vi "Decode response.vi"(8 "error in":errorcluster, 10 "response in":string="$ID1,1.6,005842.1,1E26", 11 "F-70 parameters in":T1 {"Last updated" format="%<%d/%m/%Y %H:%M:%S>T"; "State of operation" items=["Local Off", "Local On", "Remote Off", "Remote On", "Cold head Run", "Cold head pause", "Fault Off", "Oil Fault Off"]; "Return pressure (PSIG)" scale=0.0..200.0; "Water in Tmp (°C)" scale=0.0..100.0; "Water out Tmp (°C)" scale=0.0..100.0; "He discharge Tmp (°C)" scale=0.0..100.0}) -> (0 "error out":errorcluster, 3 "F-70 parameters out":T1 {"Last updated" format="%<%d/%m/%Y %H:%M:%S>T"; "State of operation" items=["Local Off", "Local On", "Remote Off", "Remote On", "Cold head Run", "Cold head pause", "Fault Off", "Oil Fault Off"]; "Return pressure (PSIG)" scale=0.0..200.0; "Water in Tmp (°C)" scale=0.0..100.0; "Water out Tmp (°C)" scale=0.0..100.0; "He discharge Tmp (°C)" scale=0.0..100.0})   [LabVIEW 2021, in "F-70 driver.lvlib"]
doc: "Process response message and updates F-70 properties cluster by values and states.\n\nErrors:\nUnknown or unexpected comunication error occured -› Sent command, checksum or format of response is incorrect.\nInvalid command code -› Compressor received invalid message."
uses:
  <instrlib>/F-70 driver/F-70 driver.lvlib
  <instrlib>/F-70 driver/public/F-70 parameters.ctl
  <instrlib>/F-70 driver/public/Commands.ctl
  <vilib>/Utility/error.llb/Error Cluster From Error Code.vi
  <vilib>/ErrorRing/Error Ring.xnode
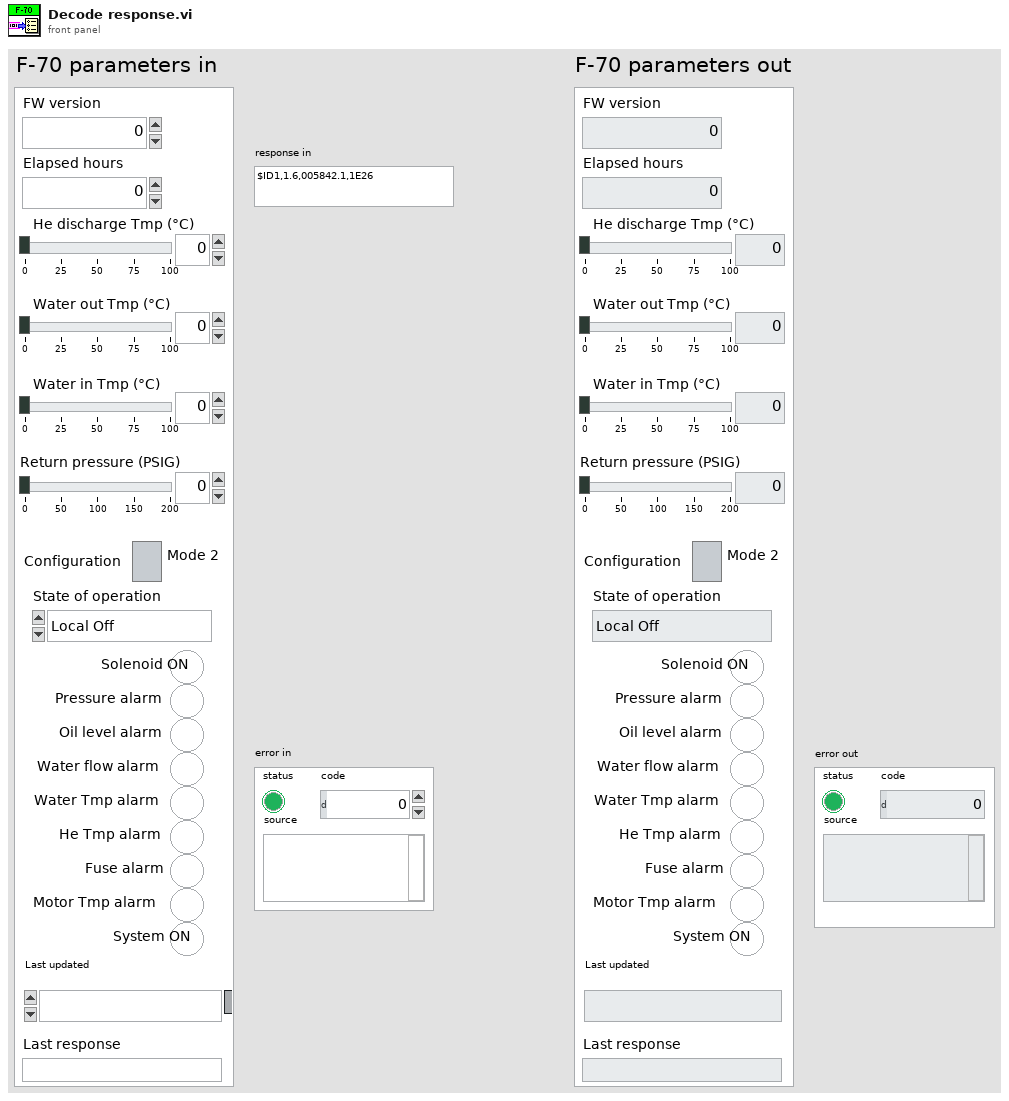
[diagram p1: front panel]
types:
  T1 = typedef "F-70 driver.lvlib/F-70 parameters.ctl" = cluster{"FW version":dbl, "Elapsed hours":dbl, "He discharge Tmp (°C)":dbl, "Water out Tmp (°C)":dbl, "Water in Tmp (°C)":dbl, "Return pressure (PSIG)":dbl, "Configuration":bool, "State of operation":u16, "Solenoid ON":bool, "Pressure alarm":bool, "Oil level alarm":bool, "Water flow alarm":bool, "Water Tmp alarm":bool, "He Tmp alarm":bool, "Fuse alarm":bool, "Motor Tmp alarm":bool, "System ON":bool, "Last updated":timestamp, "Last response":string}
  T2 = typedef "F-70 driver.lvlib/Commands.ctl" = enum16{"TEA", "PRA", "STA", "ID1", "ON1", "RS1", "CHP", "OFF", "CHR", "POF", "TE1", "TE2", "TE3", "TE4", "PR1", "PR2", "???"}
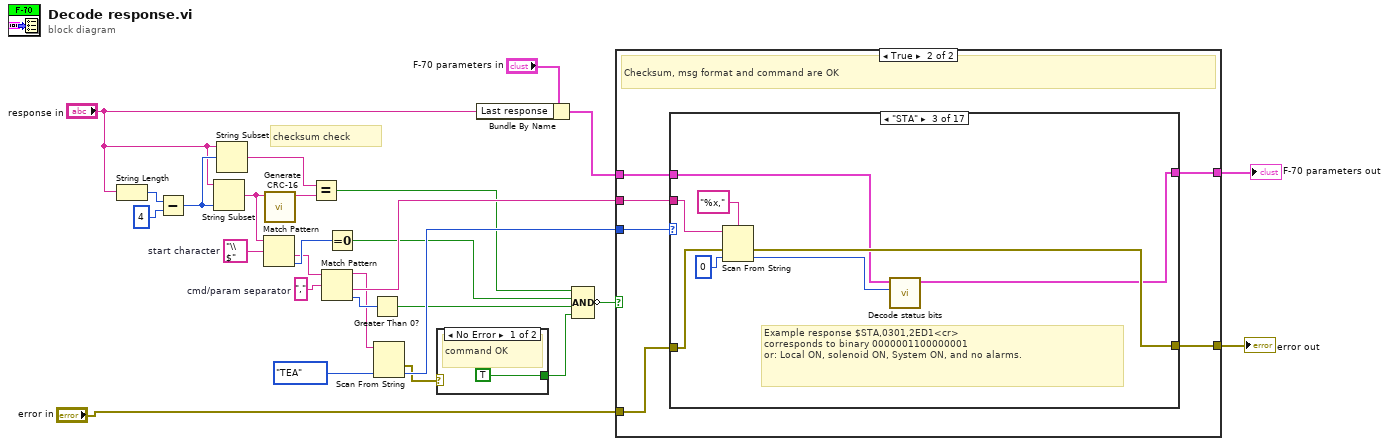
[diagram p0: block diagram]
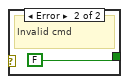
[diagram p2: hidden frame]
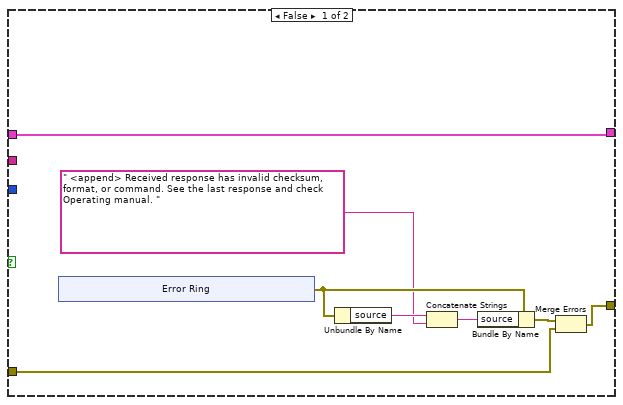
[diagram p3: hidden frame]
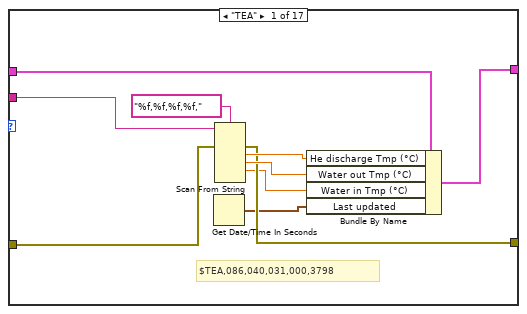
[diagram p4: hidden frame]
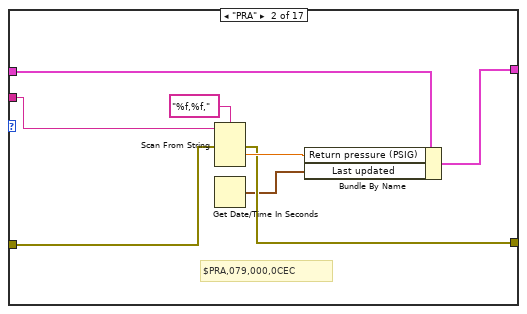
[diagram p5: hidden frame]
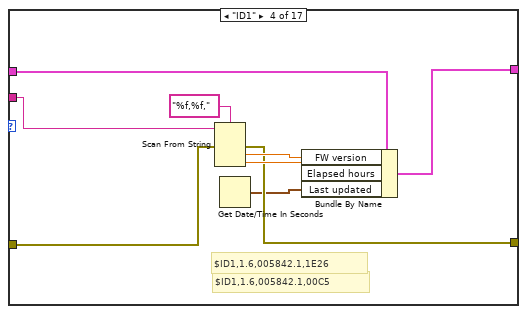
[diagram p6: hidden frame]
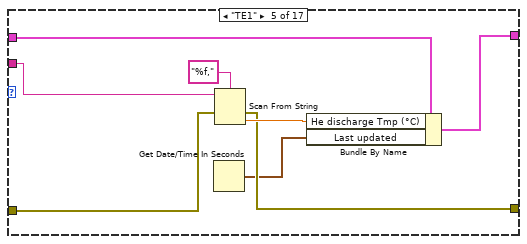
[diagram p7: hidden frame]
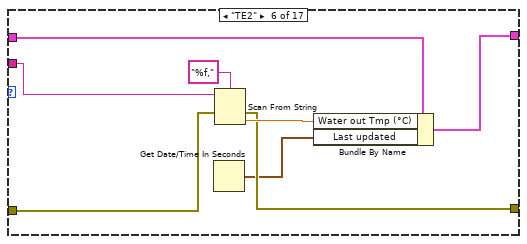
[diagram p8: hidden frame]
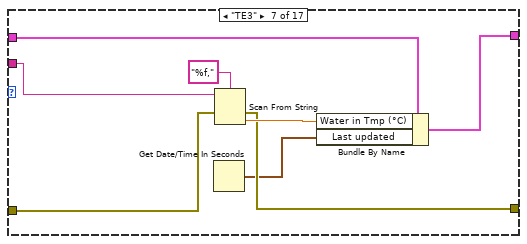
[diagram p9: hidden frame]
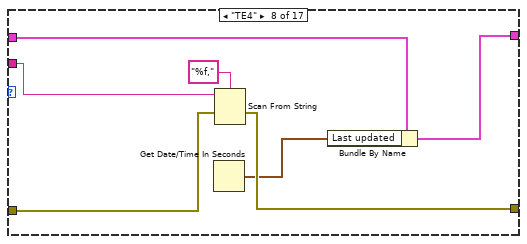
[diagram p10: hidden frame]
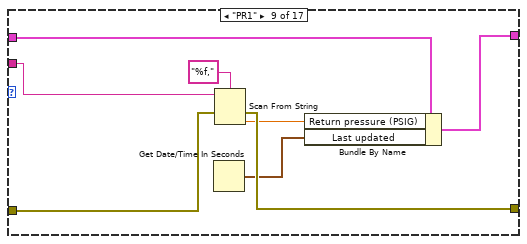
[diagram p11: hidden frame]
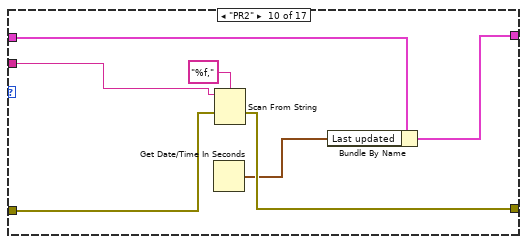
[diagram p12: hidden frame]
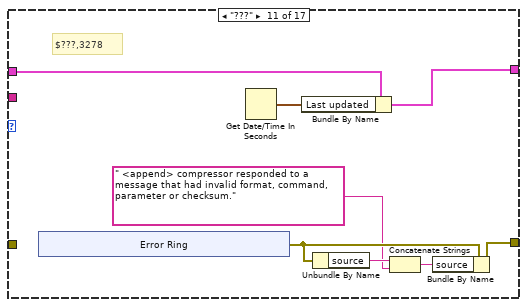
[diagram p13: hidden frame]
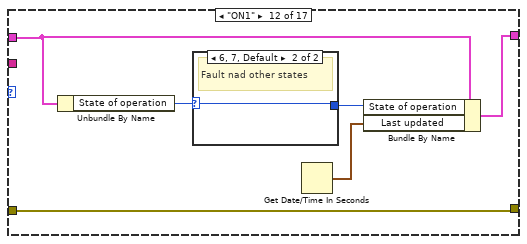
[diagram p14: hidden frame]
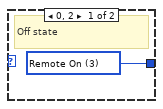
[diagram p15: hidden frame]
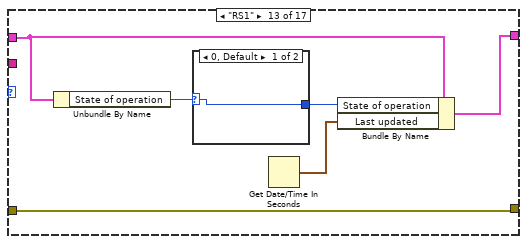
[diagram p16: hidden frame]
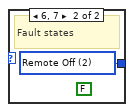
[diagram p17: hidden frame]
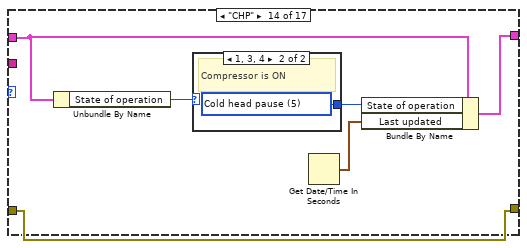
[diagram p18: hidden frame]
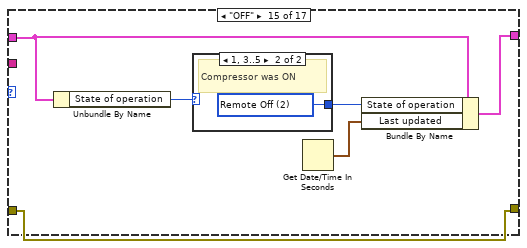
[diagram p20: hidden frame]
diagram:
  w16 = ","  # cmd/param separator
  w20 = "\\$"  # start character
  # "checksum check"
  n1 = String Length(string="response in") -> (length=w26:i32)
  n2 = Subtract(x=w26, y=4) -> (x-y=w24:i32)
  n3 = String Subset(string="response in", length (rest)=w24) -> (substring=w21:string)  [unwired: 1 in]
  n4 = String Subset(string="response in", offset (0)=w24) -> (substring=w11:string)  [unwired: 1 in]
  n5 = Match Pattern(string=w21, regular expression=w20) -> (after substring=w17:string, offset past match=w19:i32)  [unwired: 1 in, 2 out]
  n6 = call <instrlib>:"Generate CRC-16.vi"("DATA PACKET"=w21) -> ("CRC-16 H-str"=w10:string)  [unwired: 4 in, 2 out]
  n7 = Equal?(x=w11, y=w10) -> (x = y?=w8:bool)
  n8 = Match Pattern(string=w17, regular expression=w16) -> (before substring=w12:string, after substring=w15:string, offset past match=w18:i32)  [unwired: 1 in, 1 out]
  n9 = Equal To 0?(x=w19) -> (x = 0?=w4:bool)
  n10 = Greater Than 0?(x=w18) -> (x > 0?=w5:bool)
  n11 = Scan From String(input string=w12, default 1=Commands."TEA" ("Commands")) -> (error out=w1:errorcluster, output 1=w13:T2)  [unwired: 3 in, 2 out]
  n12 = case shown="No Error" w1 {
    tunnel: [TRUE FALSE] -> w3
    frame No Error {
      # "command OK"
    }
    frame Error {
      # "Invalid cmd"
    }
  }
  n13 = Bundle By Name(cluster="F-70 parameters in", "Last response"="response in") -> (w7:T1)
  n14 = Compound Arithmetic op=AND(w8, w4, w5, w3) -> (invert w9:bool)
  n15 = case shown="True" w9 {
    tunnel: [w32 w47] -> w27
    tunnel: "error in" -> [w31 w46]
    tunnel: [w33 w45] -> w22
    tunnel: w15 -> [_ w44]
    tunnel: w13 -> [_ w43]
    tunnel: w7 -> [w33 w42]
    frame False {
      n16 = xnode "Error Ring"() -> ("error out"=w35:errorcluster)
      n17 = Unbundle By Name(w35) -> ("source"=w36:string)
      n18 = Concatenate Strings(w36, " <append> Received response has invalid checksum, format, or command. See the last response and check Operating manual. " ("string")) -> (w37:string)
      n19 = Bundle By Name(cluster=w35, "source"=w37) -> (w34:errorcluster)
      n20 = Merge Errors(w34, w31) -> (w32:errorcluster)
    }
    frame True {
      # "Checksum, msg format and command are OK"
      n21 = case shown="\"STA\"" w43 {
        tunnel: [w51 w60 w71 w76 w85 w93 w101 w109 w117 w124 w133 w144 w152 w160 w168 w176 w181] -> w47
        tunnel: w46 -> [w52 w61 w72 w77 w86 w94 w102 w110 w118 w125 _ w144 w152 w160 w168 w176 w181]
        tunnel: w42 -> [w56 w64 w69 w81 w89 w97 w105 w112 w120 w127 w136 w143 w151 w159 w167 w175 w183]
        tunnel: [w53 w62 w68 w78 w87 w95 w103 w111 w119 w126 w135 w146 w154 w162 w170 w178 w182] -> w45
        tunnel: w44 -> [w48 w58 w66 w74 w83 w91 w99 w107 w114 w122 _ _ _ _ _ _ _]
        frame "TEA" {
          # "$TEA,086,040,031,000,3798"
          n22 = Get Date/Time In Seconds() -> (seconds since 1Jan1904=w50:timestamp)
          n23 = Scan From String(format string="%f,%f,%f,%f,", input string=w48, error in=w52) -> (error out=w51:errorcluster, output 1=w55:dbl, output 2=w54:dbl, output 3=w49:dbl)  [unwired: 6 in, 2 out]
          n24 = Bundle By Name(cluster=w56, "He discharge Tmp (°C)"=w55, "Water out Tmp (°C)"=w54, "Water in Tmp (°C)"=w49, "Last updated"=w50) -> (w53:T1)
        }
        frame "PRA" {
          # "$PRA,079,000,0CEC"
          n25 = Scan From String(format string="%f,%f,", input string=w58, error in=w61) -> (error out=w60:errorcluster, output 1=w63:dbl)  [unwired: 4 in, 2 out]
          n26 = Get Date/Time In Seconds() -> (seconds since 1Jan1904=w59:timestamp)
          n27 = Bundle By Name(cluster=w64, "Return pressure (PSIG)"=w63, "Last updated"=w59) -> (w62:T1)
        }
        frame "STA" {
          # "Example response $STA,0301,2ED1<cr> \ncorresponds to binary 0000001100000001 \nor: Local ON, solenoid ON, System ON, and no alarms."
          n28 = Scan From String(format string="%x,", input string=w66, error in=w72, default 1=u16 0 ("index")) -> (error out=w71:errorcluster, output 1=w67:u16)  [unwired: 1 in, 2 out]
          n29 = call <instrlib>:"Decode status bits.vi"("Status bits"=w67, "F-70 parameters in in"=w69) -> ("F-70 parameters out"=w68:T1)  [unwired: 9 in]
        }
        frame "ID1" {
          # "$ID1,1.6,005842.1,00C5"
          # "$ID1,1.6,005842.1,1E26"
          n30 = Scan From String(format string="%f,%f,", input string=w74, error in=w77) -> (error out=w76:errorcluster, output 1=w80:dbl, output 2=w79:dbl)  [unwired: 3 in, 2 out]
          n31 = Get Date/Time In Seconds() -> (seconds since 1Jan1904=w75:timestamp)
          n32 = Bundle By Name(cluster=w81, "FW version"=w80, "Elapsed hours"=w79, "Last updated"=w75) -> (w78:T1)
        }
        frame "TE1" {
          n33 = Get Date/Time In Seconds() -> (seconds since 1Jan1904=w84:timestamp)
          n34 = Scan From String(format string="%f,", input string=w83, error in=w86) -> (error out=w85:errorcluster, output 1=w88:dbl)  [unwired: 2 in, 2 out]
          n35 = Bundle By Name(cluster=w89, "He discharge Tmp (°C)"=w88, "Last updated"=w84) -> (w87:T1)
        }
        frame "TE2" {
          n36 = Get Date/Time In Seconds() -> (seconds since 1Jan1904=w92:timestamp)
          n37 = Scan From String(format string="%f,", input string=w91, error in=w94) -> (error out=w93:errorcluster, output 1=w96:dbl)  [unwired: 2 in, 2 out]
          n38 = Bundle By Name(cluster=w97, "Water out Tmp (°C)"=w96, "Last updated"=w92) -> (w95:T1)
        }
        frame "TE3" {
          n39 = Get Date/Time In Seconds() -> (seconds since 1Jan1904=w100:timestamp)
          n40 = Scan From String(format string="%f,", input string=w99, error in=w102) -> (error out=w101:errorcluster, output 1=w104:dbl)  [unwired: 2 in, 2 out]
          n41 = Bundle By Name(cluster=w105, "Water in Tmp (°C)"=w104, "Last updated"=w100) -> (w103:T1)
        }
        frame "TE4" {
          n42 = Get Date/Time In Seconds() -> (seconds since 1Jan1904=w108:timestamp)
          n43 = Scan From String(format string="%f,", input string=w107, error in=w110) -> (error out=w109:errorcluster)  [unwired: 3 in, 2 out]
          n44 = Bundle By Name(cluster=w112, "Last updated"=w108) -> (w111:T1)
        }
        frame "PR1" {
          n45 = Get Date/Time In Seconds() -> (seconds since 1Jan1904=w116:timestamp)
          n46 = Scan From String(format string="%f,", input string=w114, error in=w118) -> (error out=w117:errorcluster, output 1=w115:dbl)  [unwired: 2 in, 2 out]
          n47 = Bundle By Name(cluster=w120, "Return pressure (PSIG)"=w115, "Last updated"=w116) -> (w119:T1)
        }
        frame "PR2" {
          n48 = Get Date/Time In Seconds() -> (seconds since 1Jan1904=w123:timestamp)
          n49 = Scan From String(format string="%f,", input string=w122, error in=w125) -> (error out=w124:errorcluster)  [unwired: 3 in, 2 out]
          n50 = Bundle By Name(cluster=w127, "Last updated"=w123) -> (w126:T1)
        }
        frame "???" {
          # "$???,3278"
          n51 = xnode "Error Ring"() -> ("error out"=w132:errorcluster)
          n52 = Get Date/Time In Seconds() -> (seconds since 1Jan1904=w134:timestamp)
          n53 = Bundle By Name(cluster=w136, "Last updated"=w134) -> (w135:T1)
          n54 = Unbundle By Name(w132) -> ("source"=w130:string)
          n55 = Concatenate Strings(w130, " <append> compressor responded to a message that had invalid format, command, parameter or checksum." ("string")) -> (w131:string)
          n56 = Bundle By Name(cluster=w132, "source"=w131) -> (w133:errorcluster)
        }
        frame "ON1" {
          n57 = Unbundle By Name(w143) -> ("State of operation"=w142:u16)
          n58 = case shown="6, 7, Default" w142 {
            selector: w142 -> [_ w148]
            tunnel: [w147 w148] -> w141
            frame 0, 2 {
              w147 = u16 3 items=["Local Off", "Local On", "Remote Off", "Remote On", "Cold head Run", "Cold head pause", "Fault Off", "Oil Fault Off"] ("State of operation")
              # "Off state"
            }
            frame 6, 7, Default {
              # "Fault nad other states"
            }
          }
          n59 = Get Date/Time In Seconds() -> (seconds since 1Jan1904=w145:timestamp)
          n60 = Bundle By Name(cluster=w143, "State of operation"=w141, "Last updated"=w145) -> (w146:T1)
        }
        frame "RS1" {
          n61 = Unbundle By Name(w151) -> ("State of operation"=w150:u16)
          n62 = case shown="0, Default" w150 {
            selector: w150 -> [w155 _]
            tunnel: [w155 w156] -> w149
            frame 0, Default {
            }
            frame 6, 7 {
              w156 = u16 2 items=["Local Off", "Local On", "Remote Off", "Remote On", "Cold head Run", "Cold head pause", "Fault Off", "Oil Fault Off"] ("State of operation")
              (unwired) FALSE
              # "Fault states"
            }
          }
          n63 = Get Date/Time In Seconds() -> (seconds since 1Jan1904=w153:timestamp)
          n64 = Bundle By Name(cluster=w151, "State of operation"=w149, "Last updated"=w153) -> (w154:T1)
        }
        frame "CHP" {
          n65 = Unbundle By Name(w159) -> ("State of operation"=w158:u16)
          n66 = case shown="1, 3, 4" w158 {
            selector: w158 -> [w163 _]
            tunnel: [w163 w164] -> w157
            frame 0, Default {
              # "other states"
            }
            frame 1, 3, 4 {
              w164 = u16 5 items=["Local Off", "Local On", "Remote Off", "Remote On", "Cold head Run", "Cold head pause", "Fault Off", "Oil Fault Off"] ("State of operation")
              # "Compressor is ON"
            }
          }
          n67 = Get Date/Time In Seconds() -> (seconds since 1Jan1904=w161:timestamp)
          n68 = Bundle By Name(cluster=w159, "State of operation"=w157, "Last updated"=w161) -> (w162:T1)
        }
        frame "OFF" {
          n69 = Unbundle By Name(w167) -> ("State of operation"=w166:u16)
          n70 = case shown="1, 3..5" w166 {
            selector: w166 -> [w171 _]
            tunnel: [w171 w172] -> w165
            frame 0, Default {
            }
            frame 1, 3..5 {
              w172 = u16 2 items=["Local Off", "Local On", "Remote Off", "Remote On", "Cold head Run", "Cold head pause", "Fault Off", "Oil Fault Off"] ("State of operation")
              # "Compressor was ON"
            }
          }
          n71 = Get Date/Time In Seconds() -> (seconds since 1Jan1904=w169:timestamp)
          n72 = Bundle By Name(cluster=w167, "State of operation"=w165, "Last updated"=w169) -> (w170:T1)
        }
        frame "CHR" {
          n73 = Unbundle By Name(w175) -> ("State of operation"=w174:u16)
          n74 = case shown="0, 2" w174 {
            selector: w174 -> [w179 _]
            tunnel: [w179 w180] -> w173
            frame 1, Default {
              # "other states"
            }
            frame 0, 2 {
              w180 = u16 4 items=["Local Off", "Local On", "Remote Off", "Remote On", "Cold head Run", "Cold head pause", "Fault Off", "Oil Fault Off"] ("State of operation")
              # "Compressor is OFF"
            }
          }
          n75 = Get Date/Time In Seconds() -> (seconds since 1Jan1904=w177:timestamp)
          n76 = Bundle By Name(cluster=w175, "State of operation"=w173, "Last updated"=w177) -> (w178:T1)
        }
        frame "POF" {
          n77 = Unbundle By Name(w183) -> ("State of operation"=w185:u16)
          n78 = case shown="5" w185 {
            selector: w185 -> [w187 _]
            tunnel: [w187 w188] -> w184
            frame 0, Default {
            }
            frame 5 {
              w188 = u16 3 items=["Local Off", "Local On", "Remote Off", "Remote On", "Cold head Run", "Cold head pause", "Fault Off", "Oil Fault Off"] ("State of operation")
            }
          }
          n79 = Get Date/Time In Seconds() -> (seconds since 1Jan1904=w186:timestamp)
          n80 = Bundle By Name(cluster=w183, "State of operation"=w184, "Last updated"=w186) -> (w182:T1)
        }
      }
    }
  }
  "error out" <- w27
  "F-70 parameters out" <- w22
